vi "tpg361_get_unit.vi"(0 "tpg361_visa":refnum<visa-resource-name>, 2 "tpg361_delay":u32=500, 3 "err_in":errorcluster, 4 "tpg361_delay 2":u32=500, 5 "tpg361_delay 3":u32=500) -> (6 "UNIT":string, 9 "err_out":errorcluster)   [LabVIEW 2019]
panel:
  out "Overall Status":bool
  out "Acknowledgement Status":bool
  out "tpg361_visa 2":refnum<visa-resource-name>
  in  "tpg361_b2r 2":u32
  in  "tpg361_b2r":u32
  # "VISA"
  # "DELAY"
  # "BYTE AT PORT"
  # "STATUS"
  # "ERROR"
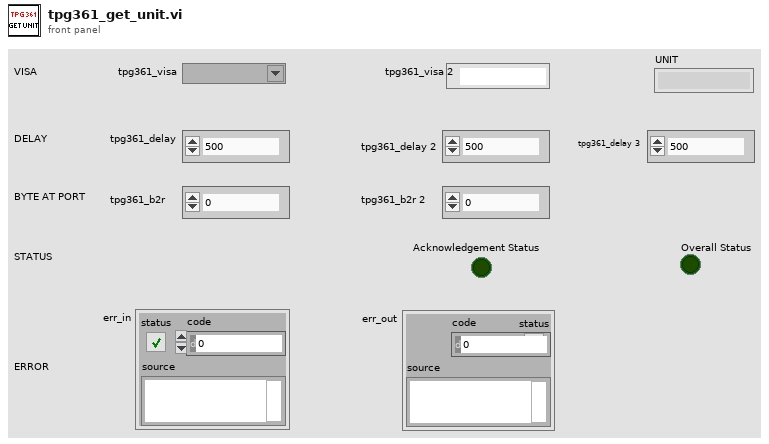
[diagram p1: front panel]
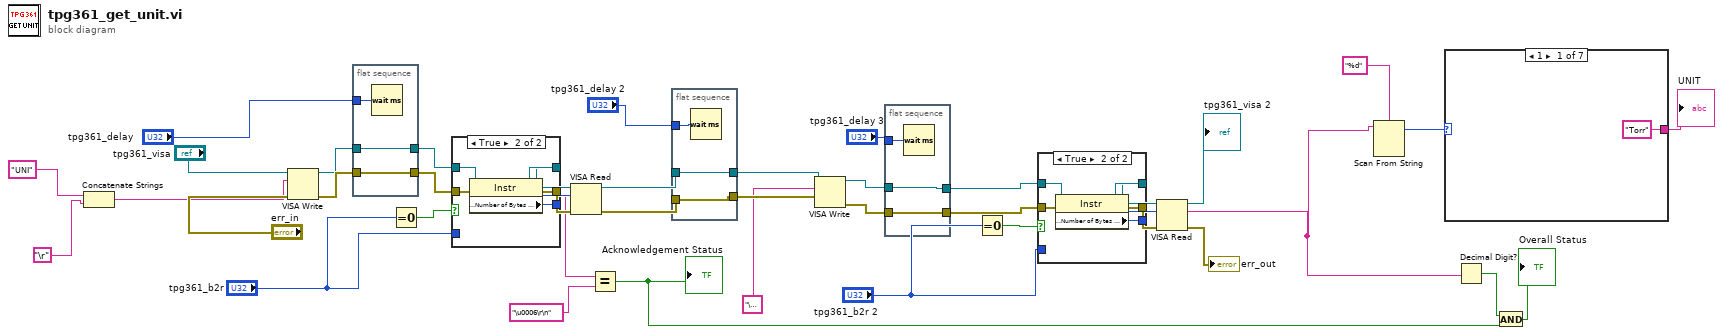
[diagram p0: block diagram]
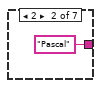
[diagram p2: hidden frame]
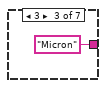
[diagram p3: hidden frame]
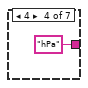
[diagram p4: hidden frame]
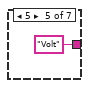
[diagram p5: hidden frame]
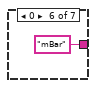
[diagram p6: hidden frame]
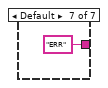
[diagram p7: hidden frame]
diagram:
  n1 = Concatenate Strings("UNI" ("string"), "\r") -> (w14:string)
  n2 = VISA Write(VISA resource name="tpg361_visa", write buffer=w14, error in (no error)="err_in") -> (VISA resource name out=w40:refnum<visa-resource-name>, error out=w42:errorcluster)  [unwired: 1 out]
  n3 = flat-sequence {
    tunnel: w42 -> [w44]
    tunnel: [w44] -> w41
    tunnel: w40 -> [w43]
    tunnel: [w43] -> w39
    tunnel: "tpg361_delay" -> [w45]
    frame #0 {
      n4 = Wait (ms)(milliseconds to wait=w45) -> ()  [unwired: 1 out]
    }
  }
  n5 = Equal To 0?(x="tpg361_b2r") -> (x = 0?=w35:bool)
  n6 = case shown="True" w35 {
    tunnel: w41 -> [w47 w53]
    tunnel: w39 -> [w48 w52]
    tunnel: [w48 w51] -> w33
    tunnel: [w47 w50] -> w32
    tunnel: [w46 w49] -> w31
    tunnel: "tpg361_b2r" -> [w46 _]
    frame False {
    }
    frame True {
      n7 = property class="Instr"(reference=w52, error in=w53) -> (reference out=w51:refnum<visa-resource-name>, error out=w50:errorcluster, "Serial Settings:Number of Bytes at Serial Port"=w49:u32)
    }
  }
  n8 = VISA Read(VISA resource name=w33, byte count=w31, error in (no error)=w32) -> (VISA resource name out=w30:refnum<visa-resource-name>, read buffer=w11:string, error out=w29:errorcluster)  [unwired: 1 out]
  n9 = Equal?(x=w11, y="\u0006\r\n") -> (x = y?=w7:bool)
  "Acknowledgement Status" <- w7
  n10 = flat-sequence {
    tunnel: [w54] -> w27
    tunnel: w30 -> [w56]
    tunnel: [w56] -> w28
    tunnel: "tpg361_delay 2" -> [w55]
    tunnel: w29 -> [w54]
    frame #0 {
      n11 = Wait (ms)(milliseconds to wait=w55) -> ()  [unwired: 1 out]
    }
  }
  n12 = VISA Write(VISA resource name=w28, write buffer="\u0005", error in (no error)=w27) -> (VISA resource name out=w20:refnum<visa-resource-name>, error out=w19:errorcluster)  [unwired: 1 out]
  n13 = flat-sequence {
    tunnel: [w58] -> w26
    tunnel: [w59] -> w25
    tunnel: w20 -> [w59]
    tunnel: w19 -> [w58]
    tunnel: "tpg361_delay 3" -> [w57]
    frame #0 {
      n14 = Wait (ms)(milliseconds to wait=w57) -> ()  [unwired: 1 out]
    }
  }
  n15 = Equal To 0?(x="tpg361_b2r 2") -> (x = 0?=w24:bool)
  n16 = case shown="True" w24 {
    tunnel: w26 -> [w61 w67]
    tunnel: w25 -> [w62 w66]
    tunnel: [w62 w65] -> w23
    tunnel: [w61 w64] -> w22
    tunnel: [w60 w63] -> w21
    tunnel: "tpg361_b2r 2" -> [w60 _]
    frame False {
    }
    frame True {
      n17 = property class="Instr"(reference=w66, error in=w67) -> (reference out=w65:refnum<visa-resource-name>, error out=w64:errorcluster, "Serial Settings:Number of Bytes at Serial Port"=w63:u32)
    }
  }
  n18 = VISA Read(VISA resource name=w23, byte count=w21, error in (no error)=w22) -> (VISA resource name out=→"tpg361_visa 2":refnum<visa-resource-name>, read buffer=w2:string, error out=→"err_out":errorcluster)  [unwired: 1 out]
  n19 = Scan From String(format string="%d", input string=w2) -> (output 1=w3:i32)  [unwired: 3 in, 3 out]
  n20 = case shown="1" w3 {
    tunnel: ["Torr" "Pascal" "Micron" "hPa" "Volt" "mBar" "ERR"] -> w5
    frame 1 {
    }
    frame 2 {
    }
    frame 3 {
    }
    frame 4 {
    }
    frame 5 {
    }
    frame 0 {
    }
    frame Default {
    }
  }
  "UNIT" <- w5
  n21 = Decimal Digit?(1:w2) -> (0:w1:bool)
  n22 = And(x=w1, y=w7) -> (x .and. y?=→"Overall Status":bool)
